vi "Set Amplifier IO Configuration.vi"(4 "error in (no error)":errorcluster, 5 "Amplifier I/O Configuration":T1={"enable amplifier fault input checking "=TRUE, "disable motor on amplifier fault event"=TRUE, "abord motion on amplifier fault event"=FALSE, "reserved"=FALSE, "reserved"=FALSE, "amplifier fault input (F:active low, T:active high)"=TRUE, "configuration Step motor control outputs (F:STEP/DIRECTION, T:+STEP/-STEP) "=FALSE, "Enable STEP output (F:active low, T:active high)"=FALSE, "Configure DIRECTION output for negative move (F:active low, T:active high)"=TRUE, "invert servo DAC output polarity "=FALSE, "amplifier enable output (F:active low, T:active high)"=FALSE, "stepper motor winding (F:FULL, T:HALF)"=FALSE, "reserved"=FALSE, "reserved "=FALSE, "reserved"=FALSE, "reserved "=FALSE, "reserved "=FALSE, "reserved "=FALSE, "reserved "=FALSE, "reserved "=FALSE, "reserved "=FALSE, "reserved "=FALSE, "reserved "=FALSE, "reserved "=FALSE, "reserved "=FALSE, "reserved "=FALSE, "reserved "=FALSE, "reserved "=FALSE, "reserved "=FALSE, "reserved"=FALSE, "reserved  "=FALSE, "reserved  "=FALSE}, 6 "Axis (1)":i32=1, 7 "VISA resource name":refnum<visa-resource-name>) -> (0 "error out":errorcluster, 3 "VISA resource name out":refnum<visa-resource-name>)   [LabVIEW 2018, in "Newport ESP301.lvlib"]
doc: "This command is used to set the amplifier I/O polarity, fault checking, and event handling for axis specified with <B>Axis (1)</B>.\n<B>NOTE:</B> If bit-0 or both bits-1 and -2 are set to zero(0) then no action will be taken by the controller."
uses:
  Newport ESP301.lvlib
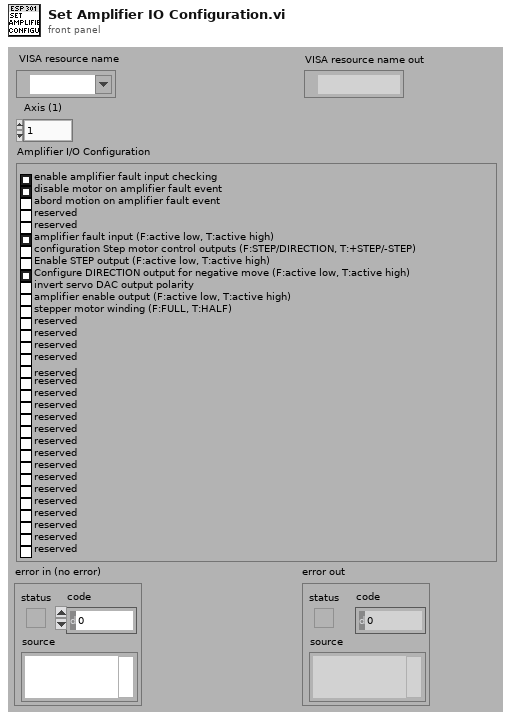
[diagram p1: front panel]
types:
  T1 = cluster{"enable amplifier fault input checking ":bool, "disable motor on amplifier fault event":bool, "abord motion on amplifier fault event":bool, "reserved":bool, "reserved":bool, "amplifier fault input (F:active low, T:active high)":bool, "configuration Step motor control outputs (F:STEP/DIRECTION, T:+STEP/-STEP) ":bool, "Enable STEP output (F:active low, T:active high)":bool, "Configure DIRECTION output for negative move (F:active low, T:active high)":bool, "invert servo DAC output polarity ":bool, "amplifier enable output (F:active low, T:active high)":bool, "stepper motor winding (F:FULL, T:HALF)":bool, "reserved":bool, "reserved ":bool, "reserved":bool, "reserved ":bool, "reserved ":bool, "reserved ":bool, "reserved ":bool, "reserved ":bool, "reserved ":bool, "reserved ":bool, "reserved ":bool, "reserved ":bool, "reserved ":bool, "reserved ":bool, "reserved ":bool, "reserved ":bool, "reserved ":bool, "reserved":bool, "reserved  ":bool, "reserved  ":bool}
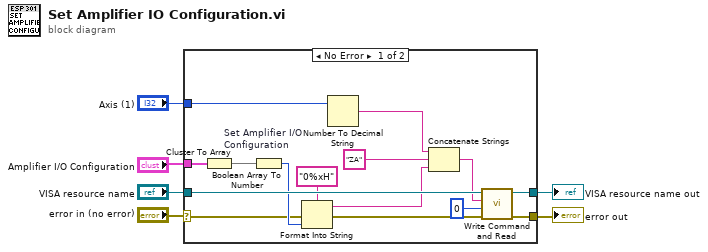
[diagram p0: block diagram]
diagram:
  n1 = case shown="No Error" "error in (no error)" {
    selector: "error in (no error)" -> [w9 w23]
    tunnel: [w20 w23] -> w6
    tunnel: "VISA resource name" -> [w21 w22]
    tunnel: [w19 w22] -> w5
    tunnel: "Axis (1)" -> [w16 _]
    tunnel: "Amplifier I/O Configuration" -> [w14 _]
    frame No Error {
      w12 = "ZA"  # Set Amplifier I/O Configuration
      n2 = Cluster To Array(cluster=w14) -> (array=w13:bool[])
      n3 = Boolean Array To Number(Boolean array=w13) -> (number=w11:u32)
      n4 = Format Into String(format string="0%xH" ("chaîne de format"), error in=w9, w11) -> (resulting string=w7:string, error out=w8:errorcluster)  [unwired: 1 in]
      n5 = Number To Decimal String(number=w16) -> (decimal integer string=w15:string)  [unwired: 1 in]
      n6 = Concatenate Strings(w15, w12, w7) -> (w18:string)
      n7 = call "Write Command and Read.vi"("error in (no error)"=w8, "Bytes to read (100)"=u32 0, "Command"=w18, "VISA resource name"=w21) -> ("error out"=w20:errorcluster, "VISA resource name out"=w19:refnum<visa-resource-name>)  [unwired: 1 in, 3 out]
    }
    frame Error {
    }
  }
  "error out" <- w6
  "VISA resource name out" <- w5
